vi "Double FFT Mesurament (Max Bin detection - Control - Init Wave&Window - Snapshot - SingleFFT) test.vi"() -> ()   [LabVIEW 2014]
uses:
  <vilib>/Platform/TimedLoop/XDataNode/timing_clust.ctl
  <vilib>/Platform/TimedLoop/XDataNode/nitl_modes.ctl
  <vilib>/Platform/TimedLoop/XDataNode/wakeup.ctl
  <vilib>/rvi/Analysis/measure/FFT/simModelSupport/niFPGA FFT Streaming Sim Properties.ctl
  <vilib>/rvi/Analysis/measure/FFT/simModelSupport/niFPGA FFT Sim Stream Group Properties.ctl
  <vilib>/rvi/Analysis/measure/FFT/simModelSupport/niFPGA FFT Sim Types.ctl
  <vilib>/rvi/Analysis/measure/FFT/simModelSupport/niFpgaFFTSimArithmeticProperties.ctl
  <vilib>/rvi/Analysis/measure/FFT/simModelSupport/niFpgaFFTSimDfxp.ctl
  <vilib>/fxp/LVFixedPointQuantizationPolicyTypeDef.ctl
  <vilib>/rvi/Analysis/measure/FFT/XNode/niFpgaFFTButterflyDelays.ctl
  <vilib>/rvi/Emulation/niFpgaSctlEmulationGetInTimedLoop.vi
  <vilib>/rvi/Emulation/niFpgaEmulationReportErrorSimple.vi
  <vilib>/rvi/Emulation/niFpgaGetClockAttributes.vi
  <vilib>/rvi/Emulation/niFpgaCriticalErrorInLSC.vi
  <vilib>/rvi/Emulation/niFpgaEmulationIsFPGAContextNoSignature.vi
  <vilib>/rvi/DataTransferAndStorage/Container/Common/niFpgaContainerGetUniqueNameForEmu.vi
  <vilib>/rvi/Memory/Memory_Emulation/niFpgaMemoryEmulationCacheClearOnFirstRun.vi
  <vilib>/rvi/Memory/Memory_Emulation/nirvimemoryEmulationManagerCache_MakeExclusive.vi
  <vilib>/rvi/Memory/Memory_Emulation/niFpgaMemoryEmulationValidateCache.vi
  <vilib>/rvi/Memory/Memory_Emulation/nirvimemoryEmulationManagerCache_InsertValue.vi
  <vilib>/Utility/error.llb/Clear Errors.vi
  <vilib>/rvi/Memory/Memory_Emulation/nirvimemoryEmulationManagerCache_ReleaseExclusive.vi
  <vilib>/rvi/Memory/Memory_Emulation/nirvimemoryEmulationManagerCache_GetValue.vi
  <vilib>/rvi/Memory/Memory_Emulation/nirvimemoryEmulationManagerCache_SetValue.vi
  <vilib>/rvi/Emulation/niFpgaProcessEmulError.vi
  <vilib>/rvi/errors/niFpgaSetErrorForExecOnDevCompSimple.vi
  <vilib>/rvi/eio/common/nirviEmuReportErrorAndStop.vi
  <vilib>/rvi/FIFO/Fifo_Resource/nirvififoEmulationSetSize.vi
  <vilib>/rvi/FIFO/Fifo_Resource/nirviFifoEmulationQueueMgr.vi
  <instcachedir>/0/nirviFifoEmulationQueueMgr_E5CAEC123FF24DC58D834DCA3CDAA9B5.lvgen/nirviFifoEmulationQueueMgr_E5CAEC123FF24DC58D834DCA3CDAA9B5_012.vi
  <vilib>/rvi/FIFO/Fifo_Resource/nirvififoEmulationCreateLock.vi
  <vilib>/rvi/FIFO/Fifo_Resource/nirvififoEmulationObtainLock.vi
  <vilib>/rvi/FIFO/Fifo_Resource/nirvififoEmulationReleaseLock.vi
  <vilib>/rvi/occurrence/nirviWaitOnOccurrenceBase.vi
  <vilib>/rvi/errors/nirviReportUnexpectedCaseInternalError.vi
  <vilib>/rvi/errors/nirviReportUnexpectedCaseInternalError (U32).vi
  <instcachedir>/0/nirviFifoEmulationQueueMgr_E5CAEC123FF24DC58D834DCA3CDAA9B5.lvgen/nirviFifoEmulationQueueMgr_E5CAEC123FF24DC58D834DCA3CDAA9B5_010.vi
  <vilib>/rvi/FIFO/Fifo_Resource/nirvififoEmulationDetermineInputValidOut.vi
  <vilib>/rvi/Memory/Memory_Emulation/nirvimemoryFastEmulation.vi
  <vilib>/rvi/Memory/Memory_Emulation/nirvimemoryEmulation.vi
  <vilib>/rvi/Analysis/measure/FFT/simModelSupport/niFpgaFFTSimModelStreamingCore.vi
  <vilib>/rvi/interface/RandomDataEmulation/niFpgaRandomDataHandleErrors.vi
  <vilib>/rvi/eio/common/nirviEmuTemplateMethod_errors.vi
  <vilib>/Platform/TimedLoop/XDataNode/XDataNode.xnode
  <vilib>/rvi/DataTransferAndStorage/Container/XNode/niFpgaContainer.xnode
  <vilib>/rvi/DataTransferAndStorage/Register/Emulation/niFpgaRegisterEmulation.vi
  <vilib>/rvi/FIFO/Fifo_Resource/nirvififoEmulationRead.vi
  <vilib>/rvi/FIFO/Fifo_Resource/nirvififoEmulationWrite.vi
  <vilib>/rvi/FIFO/Fifo_Resource/nirvififoEmulationGetNumberOfElementsToWrite.vi
  <vilib>/rvi/Analysis/measure/FFT/XNode/niFpgaFFT.xnode
  <vilib>/rvi/interface/RandomDataEmulation/nirviRandomDataFpgaReadWriteTemplate.vi
  <vilib>/eio/EIOMethodNode/EIOMethodNode.xnode
  <vilib>/Platform/TimedLoop/XDataNode/XDNodeRunTimeDep.lvlib
panel:
  in  "snapshot":bool
  in  "first bin":i32=4
  in  "last bin":i32=251
  in  "lower limit 2":u32=682
  in  "lower limit 1":u32=57
  in  "upper limit 2":u32=1193
  in  "upper limit 1":u32=568
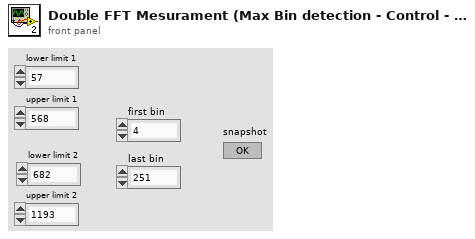
[diagram p1: front panel]
types:
  T1 = typedef "XDNodeRunTimeDep.lvlib/timing_clust.ctl" = cluster{"Expected End [f-1]":u64, "Actual End [f-1]":u64, "Finished Late? [f-1]":bool, "Expected End [i-1]":u64, "Actual End [i-1]":u64, "Finished Late? [i-1]":bool, "Expected Start [i]":u64, "Actual Start [i]":u64, "Expected Start [f]":u64, "Actual Start [f]":u64, "Source Name":string, "Structure Name":string, "Period":i64, "Deadline":i64, "Offset":i64, "Start":i64, "Priority":i32, "Timeout":i32, "Mode":T2, "Wakeup Reason":T3, "Error":errorcluster, "Source Type":string, "Secondary Source Type":string, "Global End Time":u64, "Global Start Time":u64, "Frame Duration":u64, "Iteration Duration":u64, "Assigned CPU":i32, "I/O Scan Engine Mode":u32}
  T2 = typedef "XDNodeRunTimeDep.lvlib/nitl_modes.ctl" = enum32{"No Change", "Process missed periods, maintain original phase", "Discard missed periods, maintain original phase", "Process missed periods, ignore original phase", "Discard missed periods, ignore original phase"}
  T3 = typedef "XDNodeRunTimeDep.lvlib/wakeup.ctl" = enum32{"Normal", "Aborted", "Asynchronous wakeup", "Timing source error", "Timed loop error", "Timeout"}
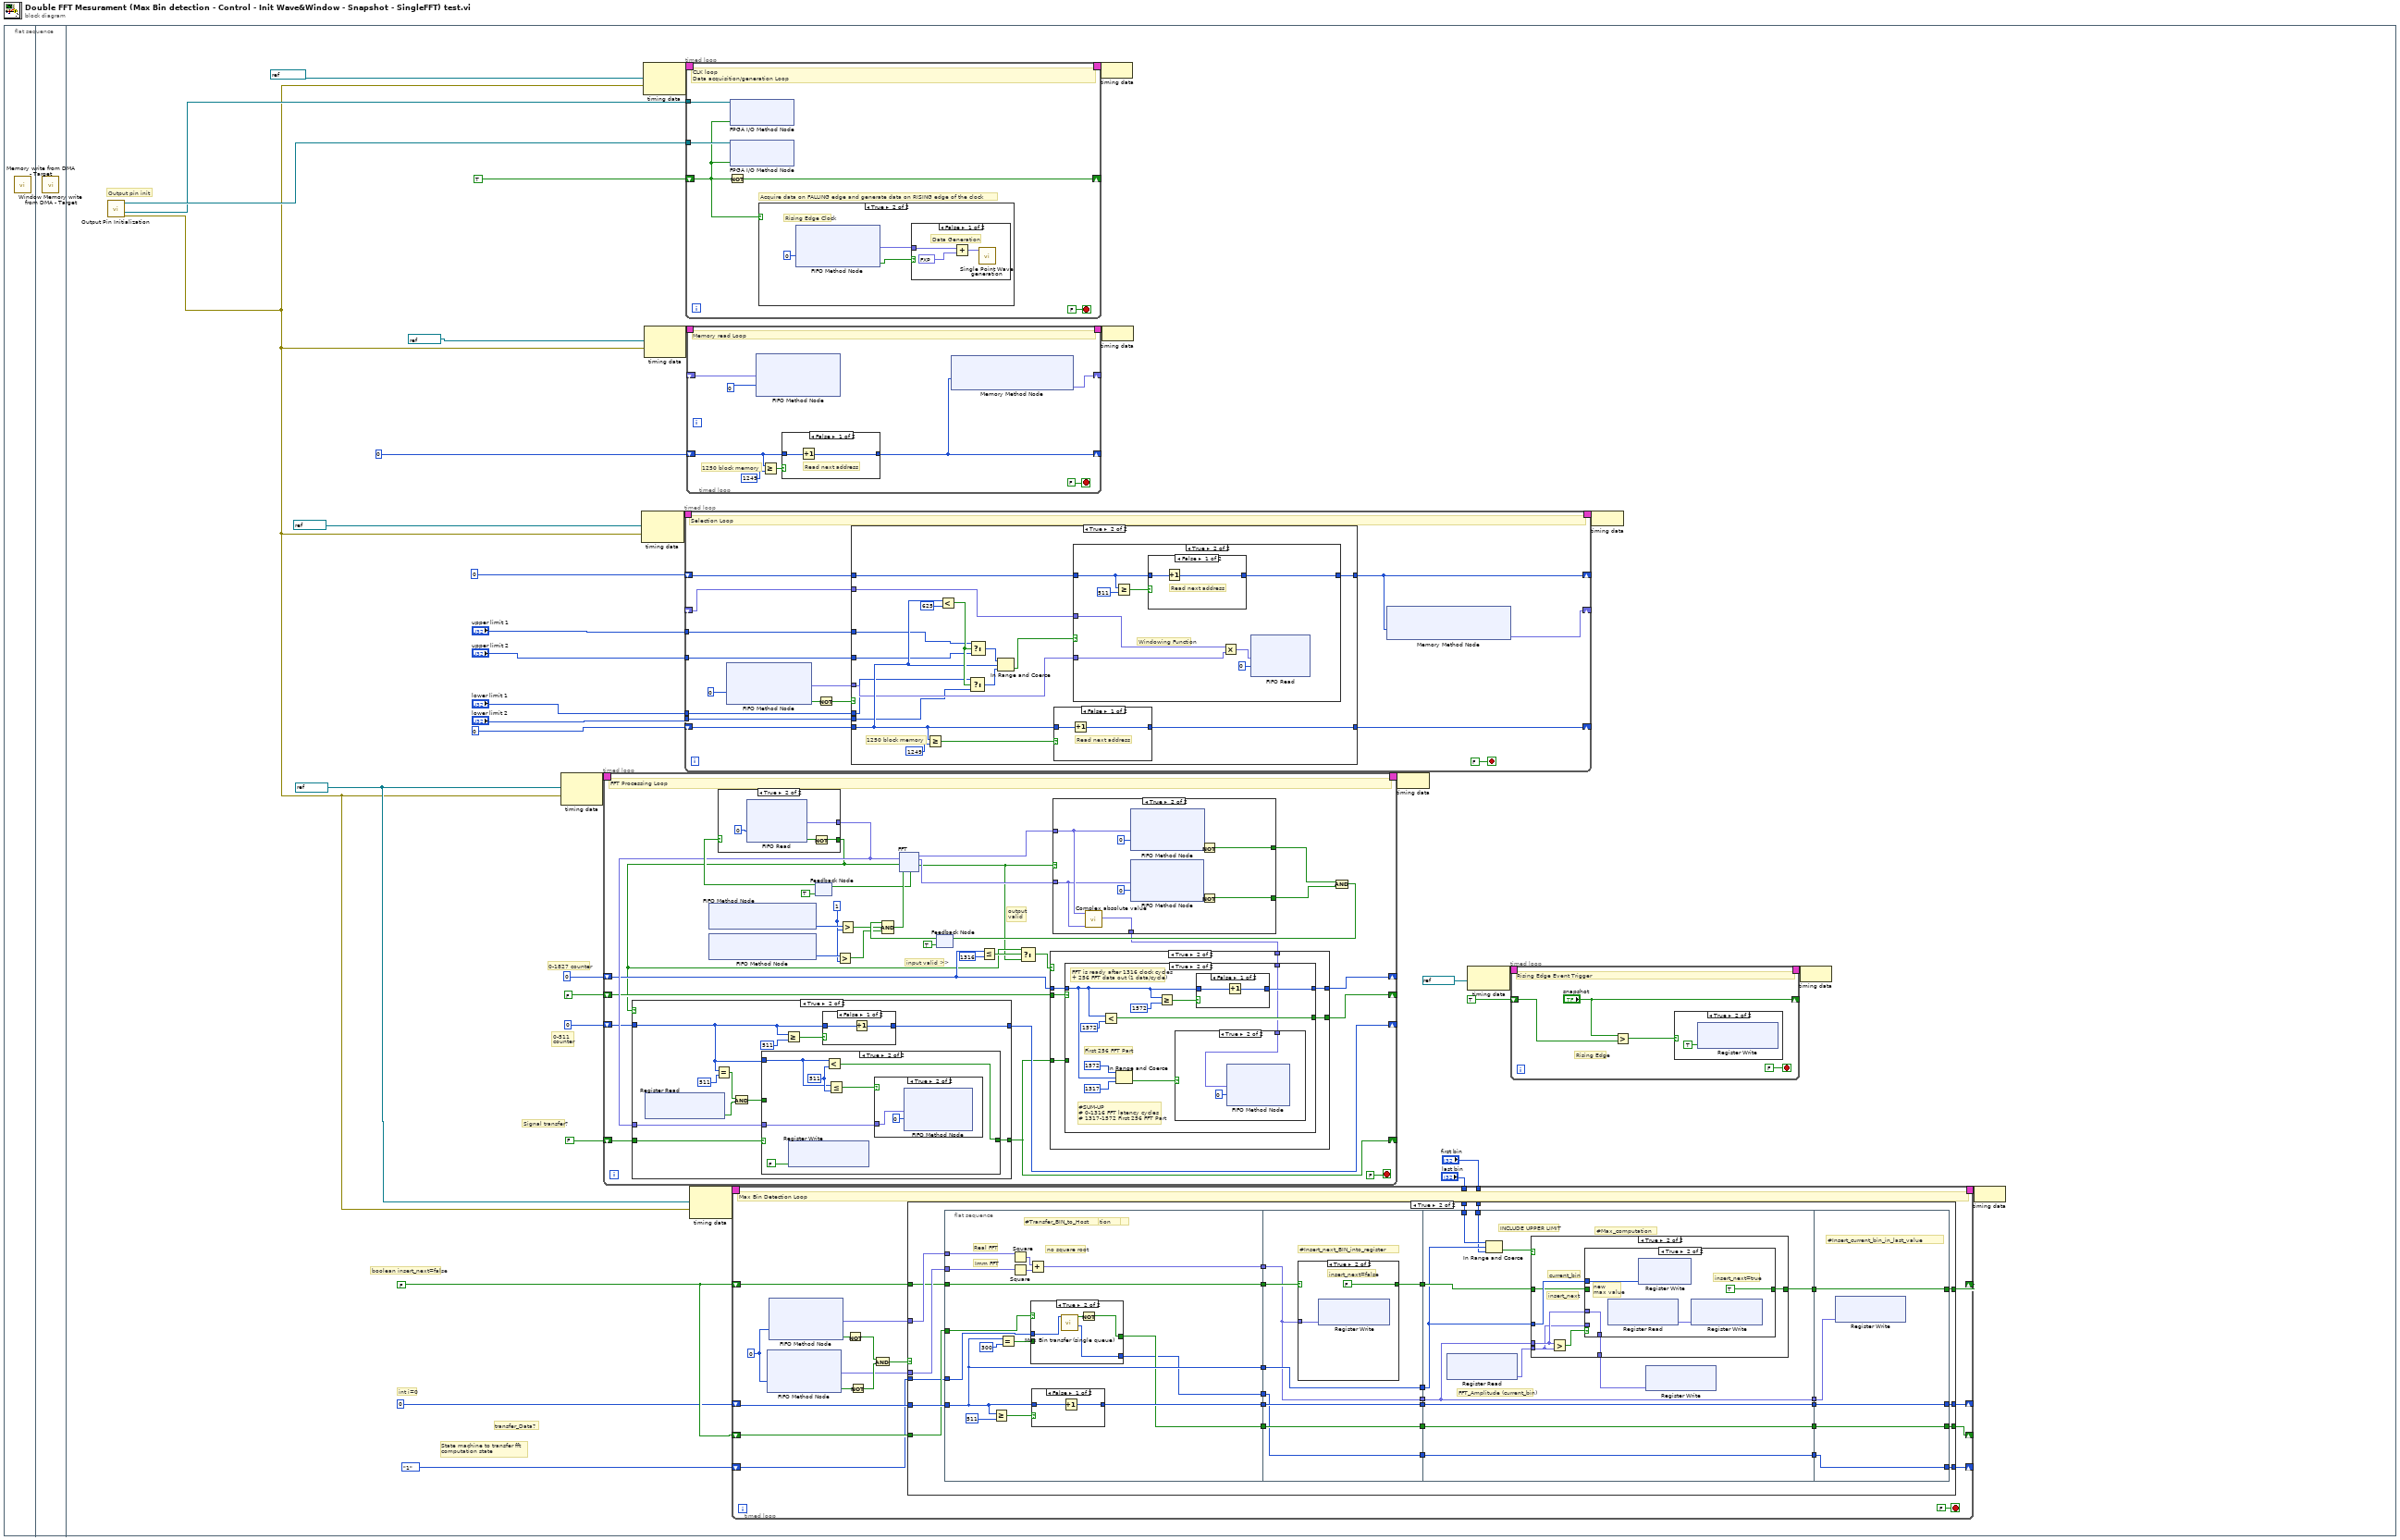
[diagram p0: block diagram]
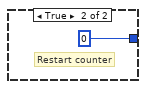
[diagram p5: hidden frame]
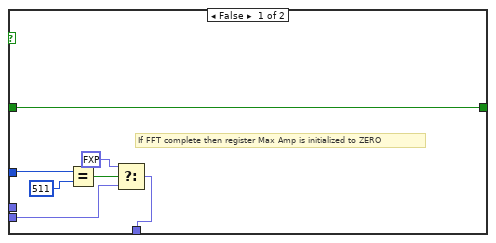
[diagram p7: hidden frame]
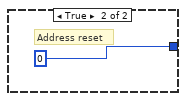
[diagram p11: hidden frame]
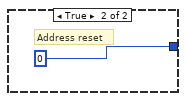
[diagram p12: hidden frame]
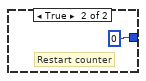
[diagram p16: hidden frame]
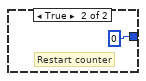
[diagram p20: hidden frame]
diagram:
  n1 = flat-sequence {
    frame #0 {
      n2 = call "Memory write from DMA - Target.vi"() -> ()  [unwired: 12 in]
    }
    frame #1 {
      n3 = call "Window Memory write from DMA - Target.vi"() -> ()  [unwired: 12 in]
    }
    frame #2 {
      w11 = FALSE
      w20 = refnum<k21> "50MHz" ("Source Name")
      # "0-1827 counter"
      # "0-511\ncounter"
      # "Signal transfer?"
      # "State machine to transfer fft\ncomputation state"
      # "transfer_Data?"
      # "int i=0"
      # "boolean insert_next=false"
      # "Output pin init"
      n4 = call "Output Pin Initialization.vi"() -> ("error out"=w19:errorcluster, "I/O Out Clock DAC (pin16)"=w23:refnum<k21>, "I/O Out Clock ADC (pin17)"=w24:refnum<k21>)  [unwired: 8 in]
      n5 = node-c288(w20, w19) -> (w34:T1)
      n6 = timed-loop {
        timing: w34 -> [_]
        timing-out: [_] -> w33
        shift-right: [w247] -> _
        shift-left: FALSE -> [w250]
        shift-right: [w251] -> _
        shift-left: i16 0 -> [w248]
        shift-right: [w246] -> _
        shift-left: FALSE -> [w245]
        shift-right: [w244] -> _
        shift-left: i16 0 -> [w241]
        stop <- FALSE stop-if-true
        w254 = u32 1 ("y")
        # "output\nvalid"
        # "input valid >>"
        # "FFT Processing Loop"
        n7 = xnode ("FIFO Method Node")() -> ("Number of Elements to Write"=w256:u32)  [unwired: 1 in, 1 out]
        n8 = xnode ("FIFO Method Node")() -> ("Number of Elements to Write"=w255:u32)  [unwired: 1 in, 1 out]
        n9 = feedback #1(TRUE ("ready for input")) -> (w268:bool)
        n10 = case shown="True" w268 {
          tunnel: [FALSE w360] -> w239
          tunnel: [fxp<+/-,12,12> 0.0 ("Element") w357] -> w249
          frame False {
            # "RMS is not ready for new input"
          }
          frame True {
            n11 = xnode ("FIFO Read")("Timeout"=0) -> ("Element"=w357:fxp<+/-,12,12>, "Timed Out?"=w359:bool)  [unwired: 1 in, 1 out]
            n12 = Not(x=w359) -> (.not. x?=w360:bool)
          }
        }
        n13 = case shown="True" w239 {
          tunnel: w248 -> [w295 w300]
          tunnel: [w295 w304] -> w251
          tunnel: w250 -> [w294 w298]
          tunnel: [w294 w299] -> w247
          tunnel: w249 -> [_ w297]
          frame False {
          }
          frame True {
            n14 = xnode ("Register Read")() -> ("Data"=w296:bool)  [unwired: 1 in, 1 out]
            n15 = Equal?(x=w300, y=i16 511) -> (x = y?=w303:bool)
            n16 = And(x=w303, y=w296) -> (x .and. y?=w301:bool)
            n17 = case shown="True" w298 {
              tunnel: w301 -> [w307 _]
              tunnel: w300 -> [_ w309]
              tunnel: [w307 w313] -> w299
              tunnel: w297 -> [_ w311]
              frame False {
              }
              frame True {
                w310 = i16 511 ("y")
                n18 = xnode ("Register Write")("Data"=FALSE) -> ()  [unwired: 1 in, 1 out]
                n19 = Less?(x=w309, y=w310) -> (x < y?=w313:bool)
                n20 = Less Or Equal?(x=w309, y=w310) -> (x <= y?=w312:bool)
                n21 = case shown="True" w312 {
                  tunnel: w311 -> [_ w314]
                  frame False {
                  }
                  frame True {
                    n22 = xnode ("FIFO Method Node")("Element"=w314, "Timeout"=0) -> ()  [unwired: 1 in, 2 out]
                  }
                }
              }
            }
            n23 = Greater Or Equal?(x=w300, y=i16 511) -> (x >= y?=w305:bool)
            n24 = case shown="False" w305 {
              tunnel: w300 -> [w317 _]
              tunnel: [w316 i16 0] -> w304
              frame False {
                n25 = Increment(x=w317) -> (x+1=w316:i16)
              }
              frame True {
                # "Restart counter"
              }
            }
          }
        }
        n26 = Greater?(x=w255, y=w254) -> (0:w252:bool)
        n27 = Greater?(x=w256, y=w254) -> (0:w253:bool)
        n28 = feedback #2(TRUE) -> (w264:bool)
        n29 = Compound Arithmetic op=AND(w264, w253, w252) -> (w263:bool)
        n30 = xnode "FFT"("real data in"=w249, "input valid"=w239, "ready for output"=w263) -> ("ready for input"=w262:bool, "real data out"=w261:fxp<+/-,22,22>, "imaginary data out"=w260:fxp<+/-,22,22>, "output valid"=w237:bool)  [unwired: 2 in, 1 out]
        n31 = feedback-in #1(w262) -> ()
        n32 = Less Or Equal?(x=w241, y=i16 1316) -> (x <= y?=w242:bool)
        n33 = Select(t=w239, s=w242, f=w237) -> (s? t:f=w238:bool)
        n34 = case shown="True" w237 {
          tunnel: w261 -> [_ w348]
          tunnel: w260 -> [_ w347]
          tunnel: [w345 w354] -> w259
          tunnel: [w345 w353] -> w258
          tunnel: [_ w346] -> w243
          frame False {
            w345 = TRUE
          }
          frame True {
            n35 = call "Complex absolute value.vi"("Im"=w347, "Re"=w348) -> ("Square Absolute Value"=w346:fxp<+,44,44>)  [unwired: 9 in]
            n36 = xnode ("FIFO Method Node")("Element"=w348, "Timeout"=0) -> ("Timed Out?"=w349:bool)  [unwired: 1 in, 1 out]
            n37 = xnode ("FIFO Method Node")("Element"=w347, "Timeout"=0) -> ("Timed Out?"=w350:bool)  [unwired: 1 in, 1 out]
            n38 = Not(x=w349) -> (.not. x?=w354:bool)
            n39 = Not(x=w350) -> (.not. x?=w353:bool)
          }
        }
        n40 = case shown="True" w238 {
          tunnel: w247 -> [_ w276]
          tunnel: [w269 w275] -> w246
          tunnel: w245 -> [w269 w274]
          tunnel: w241 -> [w270 w273]
          tunnel: [w270 w272] -> w244
          tunnel: w243 -> [_ w271]
          frame False {
          }
          frame True {
            n41 = case shown="True" w274 {
              tunnel: w276 -> [w278 _]
              tunnel: [w278 w288] -> w275
              tunnel: w273 -> [w277 w281]
              tunnel: [w277 w284] -> w272
              tunnel: w271 -> [_ w279]
              frame False {
              }
              frame True {
                # "First 256 FFT Part"
                # "#SUM-UP\n# 0-1316 FFT latency cycles\n# 1317-1572 First 256 FFT Part"
                # "FFT is ready after 1316 clock cycles\n+ 256 FFT data out (1 data/cycle)"
                n42 = Less?(x=w281, y=i16 1572) -> (x < y?=w288:bool)
                n43 = In Range and Coerce(upper limit=i16 1572, x=w281, lower limit=i16 1317 ("y")) -> (In Range?=w280:bool)  [unwired: 1 out]
                n44 = Greater Or Equal?(x=w281, y=i16 1572) -> (x >= y?=w285:bool)
                n45 = case shown="True" w280 {
                  tunnel: w279 -> [_ w290]
                  frame False {
                  }
                  frame True {
                    n46 = xnode ("FIFO Method Node")("Element"=w290, "Timeout"=0) -> ()  [unwired: 1 in, 2 out]
                  }
                }
                n47 = case shown="False" w285 {
                  tunnel: w281 -> [w292 _]
                  tunnel: [w291 i16 0] -> w284
                  frame False {
                    n48 = Increment(x=w292) -> (x+1=w291:i16)
                  }
                  frame True {
                    # "Restart counter"
                  }
                }
              }
            }
          }
        }
        n49 = Compound Arithmetic op=AND(w259, w258) -> (w257:bool)
        n50 = feedback-in #2(w257) -> ()
      }
      n51 = node-c288(refnum<k21> "50MHz" ("Source Name"), w19) -> (w32:T1)
      n52 = node-c288(refnum<k21> "100MHz" ("Source Name"), w19) -> (w38:T1)
      n53 = node-c288(refnum<k21> "50MHz" ("Source Name"), w19) -> (w36:T1)
      n54 = timed-loop {
        timing: w32 -> [_]
        timing-out: [_] -> w31
        shift-right: [w194] -> _
        shift-left: u32 0 -> [w193]
        tunnel: "upper limit 1" -> [w188]
        tunnel: "upper limit 2" -> [w187]
        tunnel: "lower limit 1" -> [w186]
        tunnel: "lower limit 2" -> [w185]
        shift-right: [w181] -> _
        shift-left: u32 0 -> [w184]
        shift-right: [w182] -> _
        shift-left: _ -> [w183]
        stop <- FALSE stop-if-true
        # "Selection Loop"
        n55 = xnode ("FIFO Method Node")("Timeout"=0) -> ("Element"=w190:fxp<+/-,12,12>, "Timed Out?"=w191:bool)  [unwired: 1 in, 1 out]
        n56 = Not(x=w191) -> (.not. x?=w192:bool)
        n57 = case shown="True" w192 {
          tunnel: [w197 w212] -> w194
          tunnel: w193 -> [w197 w207]
          tunnel: w190 -> [_ w205]
          tunnel: w188 -> [_ w204]
          tunnel: w187 -> [_ w203]
          tunnel: w186 -> [_ w202]
          tunnel: w185 -> [_ w201]
          tunnel: w184 -> [w196 w198]
          tunnel: [w196 w200] -> w181
          tunnel: w183 -> [_ w199]
          frame False {
          }
          frame True {
            # "1250 block memory"
            n58 = Greater Or Equal?(x=w207, y=u32 1249) -> (x >= y?=w213:bool)
            n59 = Less?(x=w207, y=u32 625) -> (x < y?=w208:bool)
            n60 = Select(t=w202, s=w208, f=w201) -> (s? t:f=w210:u32)
            n61 = Select(t=w204, s=w208, f=w203) -> (s? t:f=w211:u32)
            n62 = In Range and Coerce(upper limit=w211, x=w207, lower limit=w210) -> (In Range?=w206:bool)  [unwired: 1 out]
            n63 = case shown="False" w213 {
              tunnel: w207 -> [w228 _]
              tunnel: [w227 u32 0] -> w212
              frame False {
                # "Read next address"
                n64 = Increment(x=w228) -> (x+1=w227:u32)
              }
              frame True {
                # "Address reset"
              }
            }
            n65 = case shown="True" w206 {
              tunnel: w205 -> [_ w216]
              tunnel: w198 -> [w215 w221]
              tunnel: [w215 w223] -> w200
              tunnel: w199 -> [_ w219]
              frame False {
              }
              frame True {
                # "Windowing Function"
                n66 = Greater Or Equal?(x=w221, y=u32 511) -> (x >= y?=w222:bool)
                n67 = case shown="False" w222 {
                  tunnel: w221 -> [w225 _]
                  tunnel: [w224 u32 0] -> w223
                  frame False {
                    # "Read next address"
                    n68 = Increment(x=w225) -> (x+1=w224:u32)
                  }
                  frame True {
                    # "Address reset"
                  }
                }
                n69 = Multiply(x=w219, y=w216) -> (x*y=w217:fxp<+/-,12,12>)
                n70 = xnode ("FIFO Read")("Element"=w217, "Timeout"=0) -> ()  [unwired: 1 in, 2 out]
              }
            }
          }
        }
        n71 = xnode ("Memory Method Node")("Address"=w181) -> ("Data"=w182:fxp<+,8,1>)  [unwired: 1 in, 1 out]
      }
      n72 = timed-loop {
        timing: w38 -> [_]
        timing-out: [_] -> w37
        shift-right: [w388] -> _
        shift-left: TRUE -> [w386]
        tunnel: w23 -> [w390]
        tunnel: w24 -> [w387]
        stop <- FALSE stop-if-true
        # "Acquire data on FALLING edge and generate data on RISING edge of the clock"
        # "CLK loop\nData acquisition/generation Loop"
        n73 = Not(x=w386) -> (.not. x?=w388:bool)
        n74 = xnode "FPGA I/O Method Node"("FPGA I/O In"=w390, "Data"=w386) -> ()  [unwired: 1 out]
        n75 = xnode "FPGA I/O Method Node"("FPGA I/O In"=w387, "Data"=w386) -> ()  [unwired: 1 out]
        n76 = case shown="True" w386 {
          frame False {
            # "Falling Edge Clock"
            n77 = call "Single Acquisition.vi"() -> ("Out"=w392:fxp<+/-,12,12>)  [unwired: 10 in, 1 out]
            n78 = xnode ("FIFO Method Node")("Element"=w392, "Timeout"=0) -> ()  [unwired: 1 in, 2 out]
          }
          frame True {
            # "Rising Edge Clock"
            n79 = xnode ("FIFO Method Node")("Timeout"=0) -> ("Element"=w393:fxp<+/-,12,12>, "Timed Out?"=w394:bool)  [unwired: 1 in, 1 out]
            n80 = case shown="False" w394 {
              tunnel: w393 -> [w398 _]
              frame False {
                # "Data Generation"
                n81 = Add(x=w398, y=fxp<+,12,12> 2048.0) -> (x+y=w396:fxp<+/-,14,14>)
                n82 = call "Single Point Wave generation.vi"("Data To Write"=w396) -> ()  [unwired: 10 in, 1 out]
              }
              frame True {
                # "FPGA memory slow"
              }
            }
          }
        }
      }
      n83 = timed-loop {
        timing: w36 -> [_]
        timing-out: [_] -> w35
        shift-right: [w368] -> _
        shift-left: u32 0 -> [w372]
        shift-right: [w370] -> _
        shift-left: _ -> [w369]
        stop <- FALSE stop-if-true
        # "1250 block memory"
        # "Memory read Loop"
        n84 = xnode ("FIFO Method Node")("Element"=w369, "Timeout"=0) -> ()  [unwired: 1 in, 2 out]
        n85 = Greater Or Equal?(x=w372, y=u32 1249) -> (x >= y?=w374:bool)
        n86 = case shown="False" w374 {
          tunnel: w372 -> [w377 _]
          tunnel: [w376 u32 0] -> w368
          frame False {
            # "Read next address"
            n87 = Increment(x=w377) -> (x+1=w376:u32)
          }
          frame True {
            # "Address reset"
          }
        }
        n88 = xnode ("Memory Method Node")("Address"=w368) -> ("Data"=w370:fxp<+/-,12,12>)  [unwired: 1 in, 1 out]
      }
      n89 = node-c288(w20, w19) -> (w30:T1)
      n90 = timed-loop {
        shift-right: [w60] -> _
        shift-left: 0 ("Timeout") -> [w61]
        shift-right: [w58] -> _
        shift-left: w11 -> [w59]
        timing: w30 -> [_]
        timing-out: [_] -> w29
        tunnel: "last bin" -> [w56]
        tunnel: "first bin" -> [w55]
        shift-right: [w52] -> _
        shift-left: w11 -> [w53]
        shift-right: [w50] -> _
        shift-left: enum16{"1", "2", "3", "4"}."1" ("Enum") -> [w51]
        stop <- FALSE stop-if-true
        w54 = 0 ("Timeout")
        # "Max Bin Detection Loop"
        n91 = xnode ("FIFO Method Node")("Timeout"=w54) -> ("Element"=w62:fxp<+/-,22,22>, "Timed Out?"=w67:bool)  [unwired: 1 in, 1 out]
        n92 = xnode ("FIFO Method Node")("Timeout"=w54) -> ("Element"=w63:fxp<+/-,22,22>, "Timed Out?"=w68:bool)  [unwired: 1 in, 1 out]
        n93 = Not(x=w68) -> (.not. x?=w66:bool)
        n94 = Not(x=w67) -> (.not. x?=w65:bool)
        n95 = And(x=w66, y=w65) -> (x .and. y?=w64:bool)
        n96 = case shown="True" w64 {
          tunnel: w63 -> [_ w101]
          tunnel: w62 -> [_ w100]
          tunnel: w61 -> [w72 w98]
          tunnel: [w72 w85] -> w60
          tunnel: w59 -> [w71 w92]
          tunnel: [w71 w87] -> w58
          tunnel: w56 -> [_ w84]
          tunnel: w55 -> [_ w83]
          tunnel: w53 -> [w70 w82]
          tunnel: [w70 w81] -> w52
          tunnel: w51 -> [w69 w77]
          tunnel: [w69 w73] -> w50
          frame False {
            # "Data are NOT ready in Target Real FFT and Target Imm FFT FIFOs"
          }
          frame True {
            n97 = flat-sequence {
              tunnel: w101 -> [w114]
              tunnel: w100 -> [w115]
              tunnel: [w108] -> w99
              tunnel: w98 -> [w107]
              tunnel: [w113] -> w97
              tunnel: [w107] -> w94
              tunnel: [w110] -> w93
              tunnel: w92 -> [w110]
              tunnel: w82 -> [w106]
              tunnel: [w104] -> w80
              tunnel: w77 -> [w103]
              tunnel: [w102] -> w74
              tunnel: w99 -> [w130]
              tunnel: w97 -> [w133]
              tunnel: [w133] -> w96
              tunnel: w94 -> [w131]
              tunnel: w93 -> [w132]
              tunnel: [w131] -> w91
              tunnel: [w130] -> w90
              tunnel: [w129] -> w89
              tunnel: w80 -> [w128]
              tunnel: [w128] -> w79
              tunnel: [w127] -> w75
              tunnel: w74 -> [w127]
              tunnel: w96 -> [w148]
              tunnel: [w148] -> w95
              tunnel: w91 -> [w143]
              tunnel: w90 -> [w145]
              tunnel: w89 -> [w146]
              tunnel: [w145] -> w88
              tunnel: [w144] -> w86
              tunnel: w84 -> [w140]
              tunnel: w83 -> [w139]
              tunnel: w79 -> [w138]
              tunnel: [w138] -> w78
              tunnel: [w137] -> w76
              tunnel: w75 -> [w137]
              tunnel: w95 -> [w171]
              tunnel: w88 -> [w173]
              tunnel: w86 -> [w172]
              tunnel: [w172] -> w87
              tunnel: [w171] -> w85
              tunnel: [w170] -> w81
              tunnel: w78 -> [w170]
              tunnel: w76 -> [w169]
              tunnel: [w169] -> w73
              frame #0 {
                # "no square root"
                # "#Transfer_BIN_to_Host"
                # "#Iteration_Counter_Computation"
                # "#FFT_Amplitude_Computation"
                # "Imm FFT"
                # "Real FFT"
                n98 = Greater Or Equal?(x=w107, y=511) -> (x >= y?=w111:bool)
                n99 = Equal?(x=w107, y=300) -> (x = y?=w105:bool)
                n100 = Square(x=w114) -> (x^2=w117:fxp<+,43,43>)
                n101 = Square(x=w115) -> (x^2=w116:fxp<+,43,43>)
                n102 = Add(x=w117, y=w116) -> (x+y=w108:fxp<+,44,44>)
                n103 = case shown="True" w106 {
                  tunnel: w105 -> [w119 _]
                  tunnel: [w119 w122] -> w104
                  tunnel: w103 -> [w118 w121]
                  tunnel: [w118 w120] -> w102
                  frame False {
                    # "FFT Comp is NOT finished"
                  }
                  frame True {
                    n104 = call "Max Bin transfer (single queue).vi"("Enum"=w121) -> ("Next state"=w120:enum16{"1", "2", "3", "4"}, "END?"=w123:bool)  [unwired: 9 in]
                    n105 = Not(x=w123) -> (.not. x?=w122:bool)
                  }
                }
                n106 = case shown="False" w111 {
                  tunnel: w107 -> [w124 _]
                  tunnel: [w125 0 ("Timeout")] -> w113
                  frame False {
                    n107 = Increment(x=w124) -> (x+1=w125:i32)
                  }
                  frame True {
                    # "Restart counter"
                  }
                }
              }
              frame #1 {
                # "#Insert_next_BIN_into_register"
                n108 = case shown="True" w132 {
                  selector: w132 -> [w134 _]
                  tunnel: [w134 FALSE] -> w129
                  tunnel: w130 -> [_ w135]
                  frame False {
                  }
                  frame True {
                    # "insert_next=false"
                    n109 = xnode ("Register Write")("Data"=w135) -> ()  [unwired: 1 in, 1 out]
                  }
                }
              }
              frame #2 {
                # "INCLUDE UPPER LIMIT"
                # "FFT_Amplitude (current_bin)"
                # "#Max_computation"
                n110 = xnode ("Register Read")() -> ("Data"=w142:fxp<+,44,44>)  [unwired: 1 in, 1 out]
                n111 = In Range and Coerce(upper limit=w140, x=w143, lower limit=w139) -> (In Range?=w147:bool)  [unwired: 1 out]
                n112 = case shown="True" w147 {
                  tunnel: w145 -> [_ w161]
                  tunnel: w143 -> [w153 w160]
                  tunnel: w146 -> [w155 w159]
                  tunnel: [w155 w158] -> w144
                  tunnel: w142 -> [w151 w156]
                  tunnel: [w149 w157] -> w141
                  frame False {
                    # "If FFT complete then register Max Amp is initialized to ZERO"
                    n113 = Equal?(x=w153, y=511) -> (x = y?=w154:bool)
                    n114 = Select(t=fxp<+,44,44> 0.0, s=w154, f=w151) -> (s? t:f=w149:fxp<+,44,44>)
                  }
                  frame True {
                    # "insert_next"
                    # "current_bin"
                    n115 = Greater?(x=w161, y=w156) -> (0:w162:bool)
                    n116 = case shown="True" w162 {
                      tunnel: w161 -> [_ w165]
                      tunnel: w160 -> [_ w168]
                      tunnel: w159 -> [w164 _]
                      tunnel: [w164 TRUE] -> w158
                      tunnel: [w163 w165] -> w157
                      tunnel: w156 -> [w163 _]
                      frame False {
                        # "Old value is re-written"
                      }
                      frame True {
                        # "new\nmax value"
                        # "insert_next=true"
                        n117 = xnode ("Register Read")() -> ("Data"=w166:fxp<+,44,44>)  [unwired: 1 in, 1 out]
                        n118 = xnode ("Register Write")("Data"=w168) -> ()  [unwired: 1 in, 1 out]
                        n119 = xnode ("Register Write")("Data"=w166) -> ()  [unwired: 1 in, 1 out]
                      }
                    }
                  }
                }
                n120 = xnode ("Register Write")("Data"=w141) -> ()  [unwired: 1 in, 1 out]
              }
              frame #3 {
                # "#Insert_current_bin_in_last_value"
                n121 = xnode ("Register Write")("Data"=w173) -> ()  [unwired: 1 in, 1 out]
              }
            }
          }
        }
      }
      n122 = node-c288(w37) -> ()
      n123 = node-c288(w35) -> ()
      n124 = node-c288(w33) -> ()
      n125 = node-c288(refnum<k21> "50MHz" ("Source Name")) -> (w4:T1)
      n126 = timed-loop {
        timing: w4 -> [_]
        timing-out: [_] -> w3
        shift-right: ["snapshot"] -> _
        shift-left: TRUE ("snapshot") -> [w41]
        stop <- FALSE stop-if-true
        # "Rising Edge"
        # "Rising Edge Event Trigger"
        n127 = Greater?(x="snapshot", y=w41) -> (0:w39:bool)
        n128 = case shown="True" w39 {
          frame False {
          }
          frame True {
            n129 = xnode ("Register Write")("Data"=TRUE) -> ()  [unwired: 1 in, 1 out]
          }
        }
      }
      n130 = node-c288(w31) -> ()
      n131 = node-c288(w3) -> ()
      n132 = node-c288(w29) -> ()
    }
  }
